vi "servoanglesforarray.vi"() -> ()   [LabVIEW 2015]
panel:
  out "Servo2 angle":dbl
  in  "stop":bool
  out "Servo1 angle":dbl
  in  "Laser Height":dbl
  in  "Laser Pos":dbl[](array[numeric])
  in  "Route":dbl[][](array[numeric])
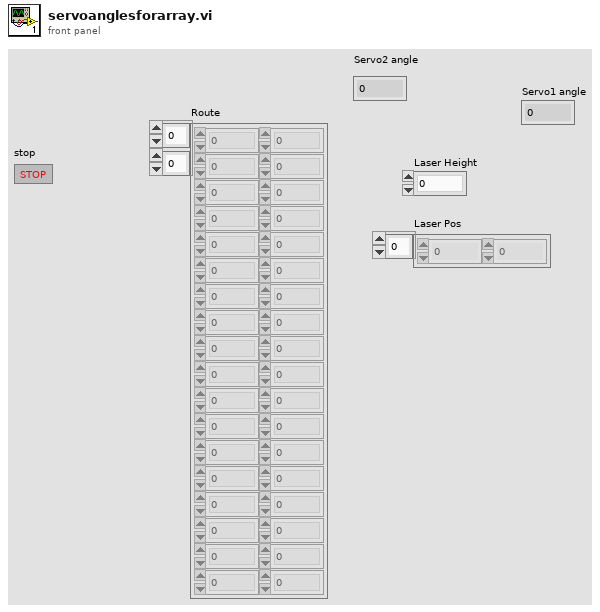
[diagram p1: front panel]
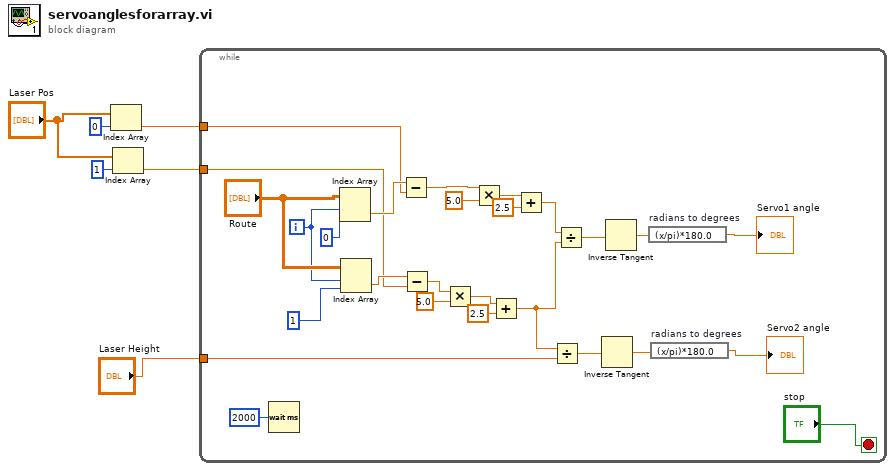
[diagram p0: block diagram]
diagram:
  n1 = Index Array(array="Laser Pos", index=0) -> (element=w3:dbl)
  n2 = Index Array(array="Laser Pos", index=1) -> (element=w2:dbl)
  n3 = while {
    tunnel: w3 -> [w28]
    tunnel: w2 -> [w26]
    tunnel: "Laser Height" -> [w10]
    i -> [w31]
    stop <- "stop" stop-if-true
    n4 = Wait (ms)(milliseconds to wait=u32 2000) -> ()  [unwired: 1 out]
    n5 = Index Array(array="Route", index (row)=w31, index (col)=0 ("disabled index (col)")) -> (element=w29:dbl)
    n6 = Index Array(array="Route", index (row)=w31, index (col)=1 ("disabled index (col)")) -> (element=w27:dbl)
    n7 = Subtract(x=w29, y=w28) -> (x-y=w22:dbl)
    n8 = Subtract(x=w27, y=w26) -> (x-y=w19:dbl)
    n9 = Multiply(x=w19, y=5.0) -> (x*y=w14:dbl)
    n10 = Multiply(x=w22, y=5.0) -> (x*y=w24:dbl)
    n11 = Add(x=w14, y=2.5) -> (x+y=w11:dbl)
    n12 = Add(x=w24, y=2.5) -> (x+y=w12:dbl)
    n13 = Divide(x=w11, y=w10) -> (x/y=w9:dbl)
    n14 = Divide(x=w12, y=w11) -> (x/y=w18:dbl)
    n15 = Inverse Tangent(1:w9) -> (0:w8:dbl)
    n16 = Inverse Tangent(1:w18) -> (0:w17:dbl)
    n17 = expression code="(x/pi)*180.0" "radians to degrees"(w17) -> (→"Servo1 angle":dbl)
    n18 = expression code="(x/pi)*180.0" "radians to degrees"(w8) -> (→"Servo2 angle":dbl)
  }
